vi "SAC-Devices Dialog (TDT).vi"(1 "Path":path) -> (8 "Canceled?":bool)   [LabVIEW 2020]
uses:
  Utility VIs/Controls/KTable/KTable.xctl
  Typedefs/SAC-Hardware Config (TDT).ctl
  PXI DAQ VIs/TDT VIs/Typedefs/TDT-Output source.ctl
  PXI DAQ VIs/TDT VIs/Typedefs/TDT-Device ID.ctl
panel:
  in  "InputTable":u16(xcontrol)
  in  "OutputTable":u16(xcontrol)
  out "Image":enum32{"None", "RX6", "RZ5", "RZ6"}(tab)
  in  "Run on":u16(ring) items=["RX6", "RZ5", "RZ6"]
  out "exit signal":bool
  in  "Cancel":bool
  in  "OK":bool
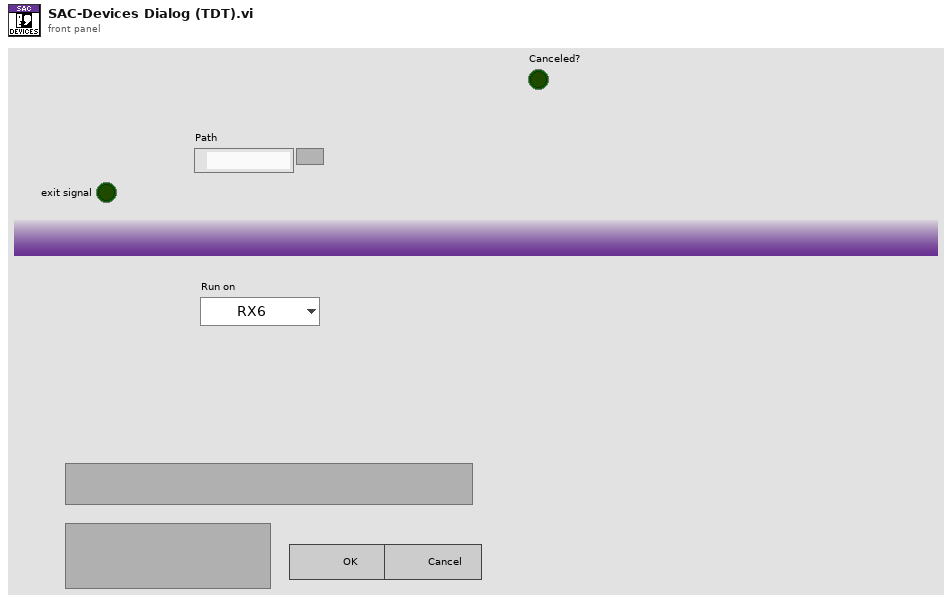
[diagram p1: front panel]
types:
  T1 = typedef "SAC-Hardware Config (TDT).ctl" = cluster{"Output":T2, "Speaker":cluster{"Channel":i32, "Primary mux":i32, "Secondary mux":i32}, "Cal mic":i32}
  T2 = typedef "TDT-Output source.ctl" = cluster{"Device":T3, "Num":i32}
  T3 = typedef "TDT-Device ID.ctl" = enum16{"None", "PA5", "RP2", "RL2", "RA16", "RV8", "RX5", "RX6", "RX7", "RX8", "RZ2", "RZ5", "RZ6"}
  T4 = cluster{string, "Channel":i32, "Primary mux":i32, "Secondary mux":i32}
  T5 = cluster{string, "Channel":i32, "Primary mux":i32, "Secondary mux":i32}[]
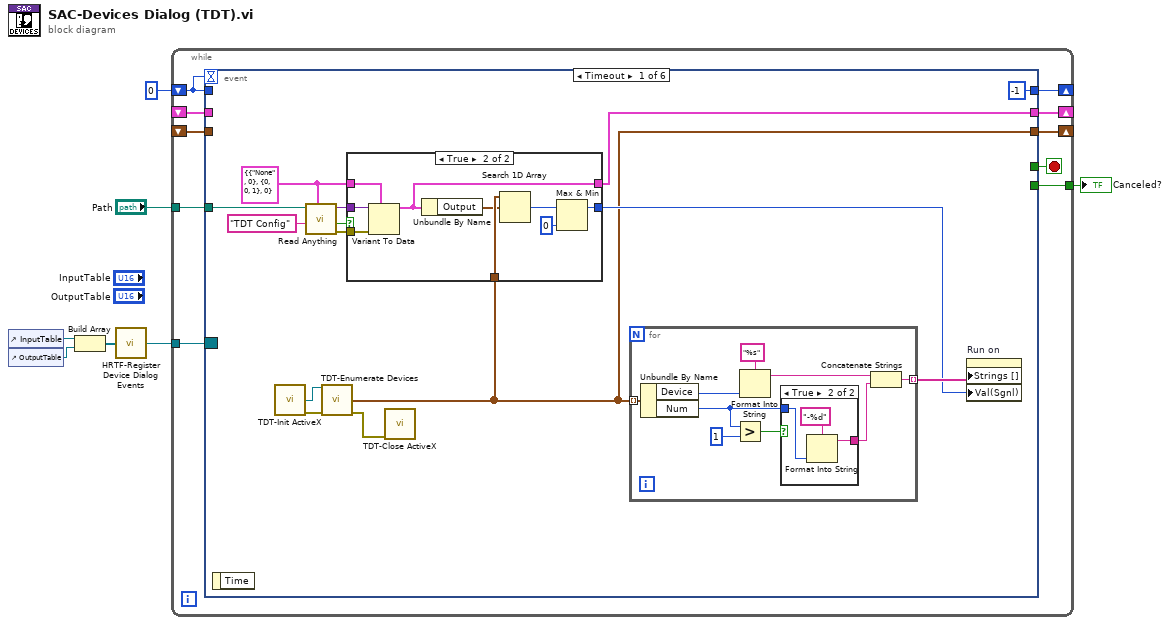
[diagram p0: block diagram]
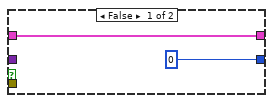
[diagram p2: hidden frame]
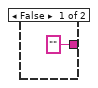
[diagram p3: hidden frame]
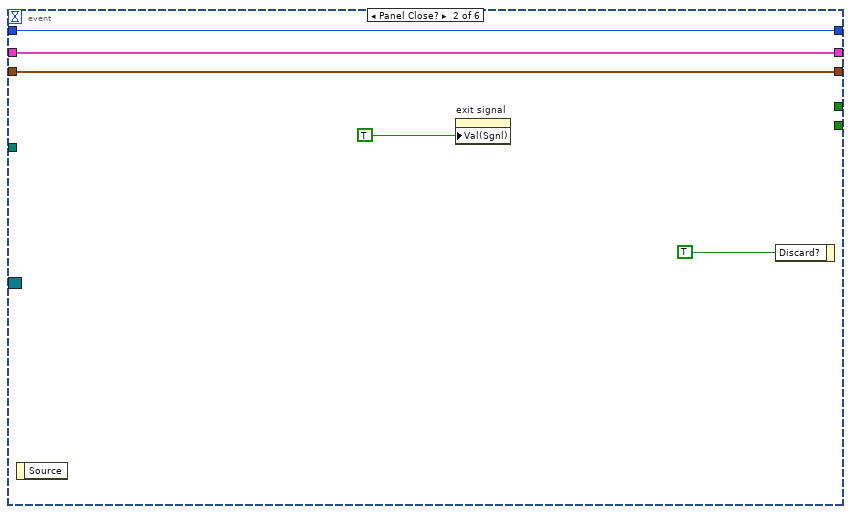
[diagram p4: hidden frame]
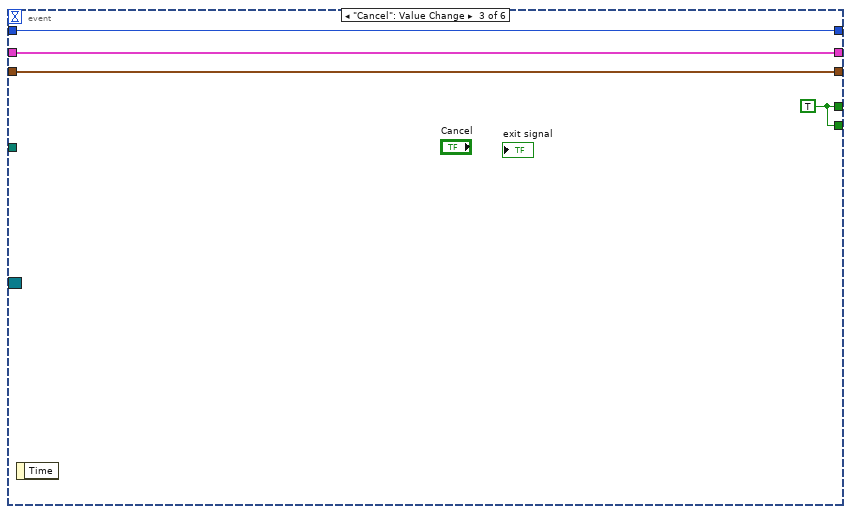
[diagram p5: hidden frame]
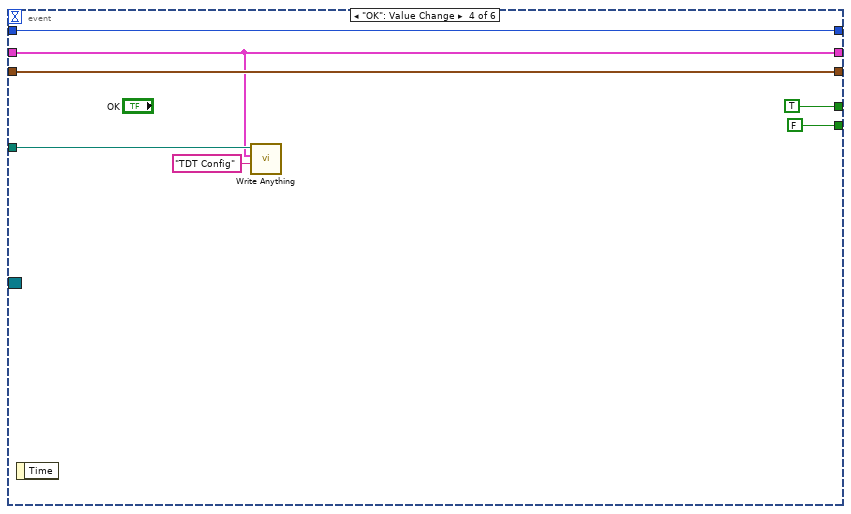
[diagram p6: hidden frame]
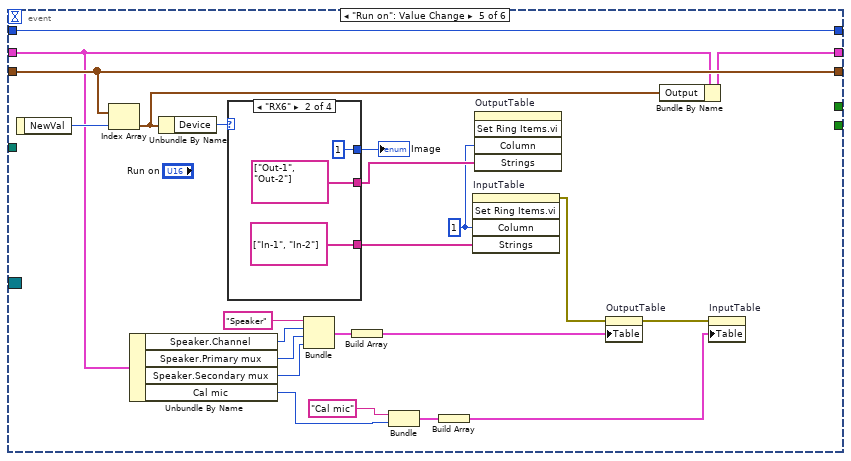
[diagram p7: hidden frame]
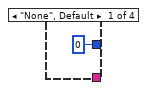
[diagram p8: hidden frame]
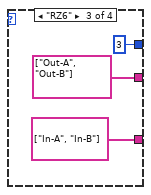
[diagram p9: hidden frame]
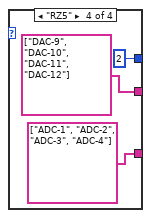
[diagram p10: hidden frame]
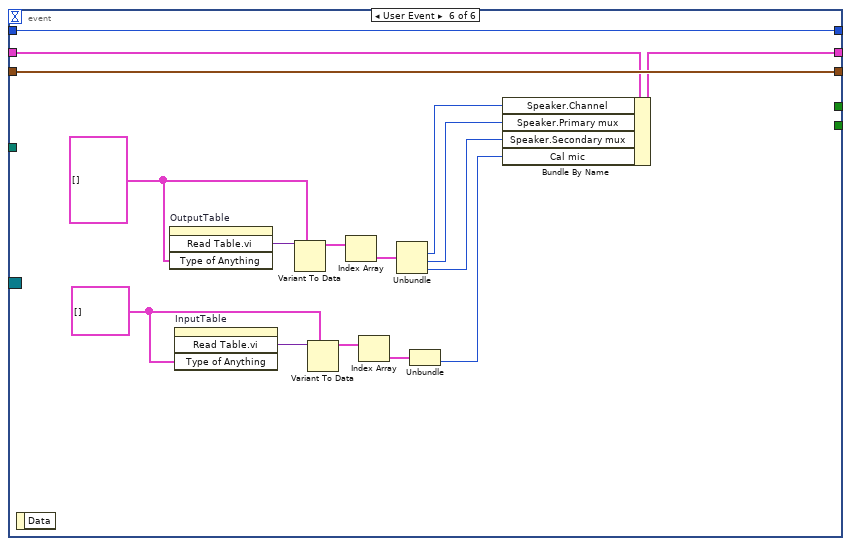
[diagram p11: hidden frame]
diagram:
  n1 = control-ref of="InputTable"() -> (w5:refnum<vi>)
  n2 = control-ref of="OutputTable"() -> (w4:refnum<vi>)
  n3 = Build Array(w5, w4) -> (w3:refnum<vi>[])
  n4 = call "HRTF-Register Device Dialog Events.vi"("Refs"=w3) -> ("Event Registration Refnum"=w2:refnum<event-registration>)  [unwired: 13 in, 1 out]
  n5 = while {
    shift-right: [w17] -> _
    shift-left: 0 -> [w14]
    tunnel: [w15] -> w6
    shift-right: [w13] -> _
    shift-left: _ -> [w12]
    tunnel: "Path" -> [w11]
    shift-right: [w10] -> _
    shift-left: _ -> [w9]
    tunnel: w2 -> [w8]
    stop <- w16 stop-if-true
    n6 = event shown="[0] Timeout" {
      selector: w8 -> [_ _ _ _ _ _]
      dyn-events: _ -> [_ _ _ _ _ _]
      timeout: w14 -> [_ _ _ _ _ _]
      tunnel: [-1 w60 w63 w69 w94 w120] -> w17
      tunnel: [_ _ w64 TRUE _ _] -> w16
      tunnel: [_ _ w64 FALSE _ _] -> w15
      tunnel: w14 -> [_ w60 w63 w69 w94 w120]
      tunnel: [w19 w57 w62 w68 w93 w119] -> w13
      tunnel: w12 -> [_ w57 w62 w68 w93 w119]
      tunnel: w11 -> [w29 _ _ w67 _ _]
      tunnel: [w22 w56 w61 w66 w74 w113] -> w10
      tunnel: w9 -> [_ w56 w61 w66 w86 w118]
      event Timeout {
        w23 = T1 {"Output"={"Device"=enum."None", "Num"=0}, "Speaker"={"Channel"=0, "Primary mux"=0, "Secondary mux"=1}, "Cal mic"=0} ("TDT")
        n7 = event-data() -> ()  [unwired: 1 in, 1 out]
        n8 = call "TDT-Init ActiveX.vi"() -> ("ZBUSx"=w20:refnum<k7>, "error out"=w21:errorcluster)  [unwired: 12 in, 2 out]
        n9 = call "Read Anything.vi"("Type of Anything"=w23, "Section Name (Name of \"Type of Anything\")"="TDT Config" ("Section Name (Name of \"Type of Anything\")"), "Path (dialog)"=w29) -> ("Error Out"=w27:errorcluster, "Found?"=w26:bool, "Anything"=w25:variant)  [unwired: 6 in]
        n10 = call "TDT-Enumerate Devices.vi"("ZBUSx In"=w20, "error in (no error)"=w21) -> ("Devices"=w19:T2[], "error out"=w18:errorcluster)  [unwired: 11 in, 1 out]
        n11 = case shown="True" w26 {
          tunnel: w27 -> [_ w42]
          tunnel: w25 -> [_ w41]
          tunnel: w23 -> [w32 w40]
          tunnel: w19 -> [_ w37]
          tunnel: [0 w36] -> w24
          tunnel: [w32 w34] -> w22
          frame False {
          }
          frame True {
            n12 = Variant To Data(error in=w42, type=w40, Variant=w41) -> (data=w34:T1)  [unwired: 1 out]
            n13 = Unbundle By Name(w34) -> ("Output"=w35:T2)
            n14 = Search 1D Array(1D array=w37, element=w35) -> (index of element=w38:i32)  [unwired: 1 in]
            n15 = Max & Min(x=w38, y=0) -> (max(x,y)=w36:i32)  [unwired: 1 out]
          }
        }
        n16 = call "TDT-Close ActiveX.vi"("error in (no error)"=w18) -> ()  [unwired: 14 in, 1 out]
        n17 = for {
          tunnel: w19 -> [w51] mode=indexing
          tunnel: [w45] -> w30 mode=indexing
          n18 = Unbundle By Name(w51) -> ("Device"=w43:T3, "Num"=w46:i32)
          n19 = Greater?(x=w46, y=1) -> (0:w47:bool)
          n20 = Format Into String(format string="%s", w43) -> (resulting string=w49:string)  [unwired: 2 in, 1 out]
          n21 = case shown="True" w47 {
            tunnel: w46 -> [_ w54]
            tunnel: ["" w53] -> w44
            frame False {
            }
            frame True {
              n22 = Format Into String(format string="-%d", w54) -> (resulting string=w53:string)  [unwired: 2 in, 1 out]
            }
          }
          n23 = Concatenate Strings(w49, w44) -> (w45:string)
        }
        n24 = property on="Run on" class="Ring (strict)"("Strings []"=w30, "Val(Sgnl)"=w24) -> ()  [unwired: 2 in, 2 out]
      }
      event Panel Close? {
        n25 = event-data() -> ()  [unwired: 1 in, 1 out]
        n26 = property on="exit signal" class="Bool (strict)"("Val(Sgnl)"=TRUE ("Value (Signaling)")) -> ()  [unwired: 2 in, 2 out]
        n27 = event-data("Discard?"=TRUE) -> ()  [unwired: 1 in, 1 out]
      }
      event "Cancel": Value Change {
        w64 = TRUE
        n28 = event-data() -> ()  [unwired: 1 in, 1 out]
      }
      event "OK": Value Change {
        n29 = event-data() -> ()  [unwired: 1 in, 1 out]
        n30 = call "Write Anything.vi"("Section Name (Name of \"Anything\")"="TDT Config" ("Section Name (Name of \"Anything\")"), "Anything"=w66, "Path (dialog)"=w67) -> ()  [unwired: 7 in, 2 out]
      }
      event "Run on": Value Change {
        w87 = 1
        n31 = event-data() -> ("NewVal"=w92:u16)  [unwired: 1 in]
        n32 = Index Array(array=w93, index=w92) -> (element=w73:T2)
        n33 = Unbundle By Name(w86) -> ("Speaker.Channel"=w84:i32, "Speaker.Primary mux"=w83:i32, "Speaker.Secondary mux"=w82:i32, "Cal mic"=w72:i32)
        n34 = Unbundle By Name(w73) -> ("Device"=w90:T3)
        n35 = case shown="\"RX6\"" w90 {
          tunnel: [0 1 3 2] -> w91
          tunnel: [_ string[] ["Out-1", "Out-2"] string[] ["Out-A", "Out-B"] string[] ["DAC-9", "DAC-10", "DAC-11", "DAC-12"]] -> w88
          tunnel: [_ string[] ["In-1", "In-2"] string[] ["In-A", "In-B"] string[] ["ADC-1", "ADC-2", "ADC-3", "ADC-4"]] -> w89
          frame "None", Default {
          }
          frame "RX6" {
          }
          frame "RZ6" {
          }
          frame "RZ5" {
          }
        }
        "Image" <- w91
        n36 = Bundle("Speaker", "Channel"=w84, "Primary mux"=w83, "Secondary mux"=w82) -> (w81:T4)  [unwired: 1 in]
        n37 = Build Array(w81) -> (w80:T5)
        n38 = Bundle("Cal mic", "Cal mic"=w72) -> (w77:cluster{string, "Cal mic":i32})  [unwired: 1 in]
        n39 = Build Array(w77) -> (w76:cluster{string, "Cal mic":i32}[])
        n40 = invoke on="InputTable" class="KTable (strict)" method="Set Ring Items.vi"("Column"=w87, "Strings"=w89) -> (error out=w79:errorcluster)  [unwired: 3 in, 4 out]
        n41 = invoke on="OutputTable" class="KTable (strict)" method="Set Ring Items.vi"("Column"=w87, "Strings"=w88) -> ()  [unwired: 3 in, 5 out]
        n42 = property on="OutputTable" class="KTable (strict)"(error in=w79, "Table"=w80) -> (error out=w75:errorcluster)  [unwired: 1 in, 1 out]
        n43 = Bundle By Name(cluster=w86, "Output"=w73) -> (w74:T1)
        n44 = property on="InputTable" class="KTable (strict)"(error in=w75, "Table"=w76) -> ()  [unwired: 1 in, 2 out]
      }
      event User Event {
        w106 = cluster{string, i32}[] []
        w116 = cluster{string, i32, i32, i32}[] []
        n45 = event-data() -> ()  [unwired: 1 in, 1 out]
        n46 = invoke on="OutputTable" class="KTable (strict)" method="Read Table.vi"("Type of Anything"=w116) -> ("Read Table.vi"=w117:variant)  [unwired: 3 in, 3 out]
        n47 = invoke on="InputTable" class="KTable (strict)" method="Read Table.vi"("Type of Anything"=w106) -> ("Read Table.vi"=w107:variant)  [unwired: 3 in, 3 out]
        n48 = Variant To Data(type=w116, Variant=w117) -> (data=w115:cluster{string, i32, i32, i32}[])  [unwired: 1 in, 1 out]
        n49 = Variant To Data(type=w106, Variant=w107) -> (data=w109:cluster{string, i32}[])  [unwired: 1 in, 1 out]
        n50 = Index Array(array=w115) -> (element=w114:cluster{string, i32, i32, i32})  [unwired: 1 in]
        n51 = Index Array(array=w109) -> (element=w108:cluster{string, i32})  [unwired: 1 in]
        n52 = Unbundle(w114) -> (w112:i32, w111:i32, w110:i32)  [unwired: 1 out]
        n53 = Unbundle(w108) -> (w105:i32)  [unwired: 1 out]
        n54 = Bundle By Name(cluster=w118, "Speaker.Channel"=w112, "Speaker.Primary mux"=w111, "Speaker.Secondary mux"=w110, "Cal mic"=w105) -> (w113:T1)
      }
    }
  }
  "Canceled?" <- w6
